vi "cumplimiento.vi"(8 "error in (no error)":errorcluster, 11 "Prueba09 in":refnum<class "Prueba10.lvclass">) -> (0 "error out":errorcluster, 3 "Prueba09 out":refnum<class "Prueba10.lvclass">)   [LabVIEW 2019, in "Prueba10.lvclass"]
uses:
  Prueba10.lvclass
  Prueba10.lvclass/Prueba10.ctl
panel:
  out "cumpimiento":string
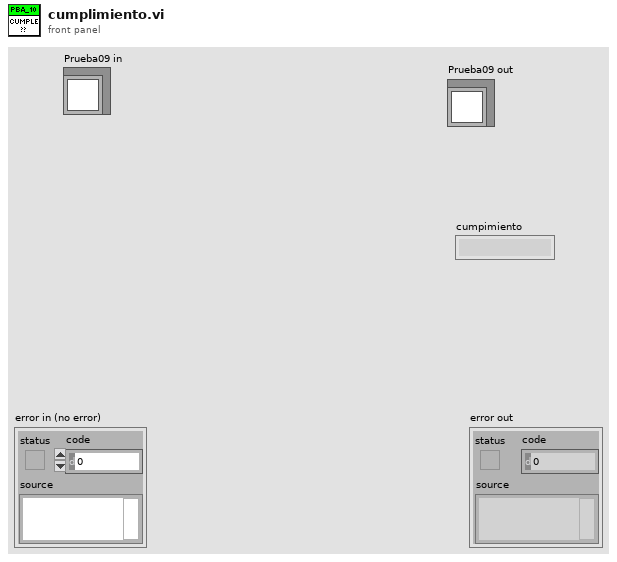
[diagram p1: front panel]
types:
  T1 = cluster{"Medido":dbl, "Error":dbl, "Ref":dbl, "Incert_exp":dbl, "Tol+":dbl, "Tol-":dbl, "fila":i32}
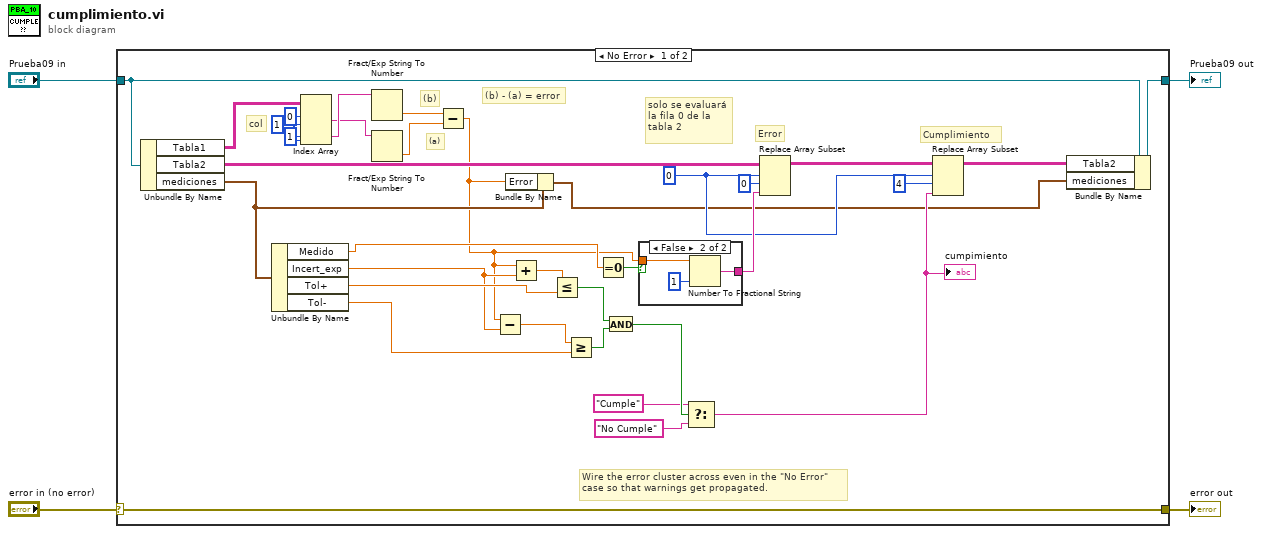
[diagram p0: block diagram]
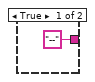
[diagram p2: hidden frame]
diagram:
  n1 = case shown="No Error" "error in (no error)" {
    selector: "error in (no error)" -> [w38 w44]
    tunnel: [w38 w44] -> w3
    tunnel: [w20 w43] -> w2
    tunnel: "Prueba09 in" -> [w18 w43]
    frame No Error {
      w13 = 1 ("disabled index (col)")
      w15 = 0 ("disabled index (col)")
      # "(b) - (a) = error"
      # "(a)"
      # "(b)"
      # "col"
      # "solo se evaluará\nla fila 0 de la \ntabla 2"
      # "Cumplimiento"
      # "Error"
      # "Wire the error cluster across even in the \"No Error\"\ncase so that warnings get propagated."
      n2 = Unbundle By Name(w18) -> ("Tabla1"=w14:string[][], "Tabla2"=w17:string[][], "mediciones"=w16:T1)
      n3 = Unbundle By Name(w16) -> ("Medido"=w21:dbl, "Incert_exp"=w29:dbl, "Tol+"=w30:dbl, "Tol-"=w28:dbl)
      n4 = Index Array(array=w14, index (row) #1=0 ("disabled index (row)"), index (col) #1=w13, index (row) #2=1 ("disabled index (row)"), index (col) #2=w13) -> (element #1=w11:string, element #2=w12:string)
      n5 = Fract/Exp String To Number(string=w12) -> (number=w10:dbl)  [unwired: 3 in, 1 out]
      n6 = Fract/Exp String To Number(string=w11) -> (number=w7:dbl)  [unwired: 3 in, 1 out]
      n7 = Subtract(x=w10, y=w7) -> (x-y=w5:dbl)
      n8 = Subtract(x=w5, y=w29) -> (x-y=w34:dbl)
      n9 = Bundle By Name(cluster=w16, "Error"=w5) -> (w6:T1)
      n10 = Add(x=w5, y=w29) -> (x+y=w37:dbl)
      n11 = Less Or Equal?(x=w37, y=w30) -> (x <= y?=w36:bool)
      n12 = Greater Or Equal?(x=w34, y=w28) -> (x >= y?=w35:bool)
      n13 = Equal To 0?(x=w21) -> (x = 0?=w22:bool)
      n14 = And(x=w36, y=w35) -> (x .and. y?=w33:bool)
      n15 = case shown="False" w22 {
        tunnel: w5 -> [_ w42]
        tunnel: ["--" w40] -> w23
        frame True {
        }
        frame False {
          n16 = Number To Fractional String(number=w42, precision (6)=i16 1) -> (F-format string=w40:string)  [unwired: 2 in]
        }
      }
      n17 = Select(t="Cumple", s=w33, f="No Cumple") -> (s? t:f=w27:string)
      "cumpimiento" <- w27
      n18 = Replace Array Subset(array=w17, new element=w23, index (row)=w15, index (col)=0 ("disabled index (col)")) -> (w25:string[][])
      n19 = Replace Array Subset(array=w25, new element=w27, index (row)=w15, index (col)=4 ("index (row)")) -> (w19:string[][])
      n20 = Bundle By Name(cluster=w18, "Tabla2"=w19, "mediciones"=w6) -> (w20:refnum<class "Prueba10.lvclass">)
    }
    frame Error {
    }
  }
  "error out" <- w3
  "Prueba09 out" <- w2
